vi "HW_Gantner_DLL paths.vi"() -> (2 "DLL paths":T1)   [LabVIEW 2016]
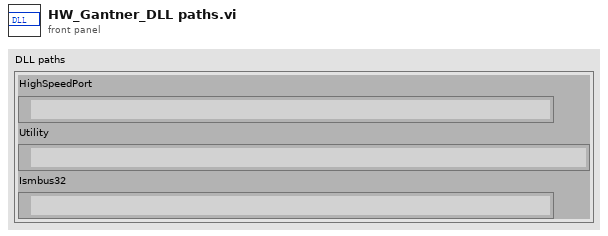
[diagram p1: front panel]
types:
  T1 = cluster{"HighSpeedPort":path, "Utility":path, "Ismbus32":path}
  T2 = enum32{"invalid app kind", "Development System", "Run Time System", "Student Edition", "Embedded LabVIEW", "Evaluation", "Custom"}
  T3 = cluster{"appended path":path, "appended path":path, "appended path":path}
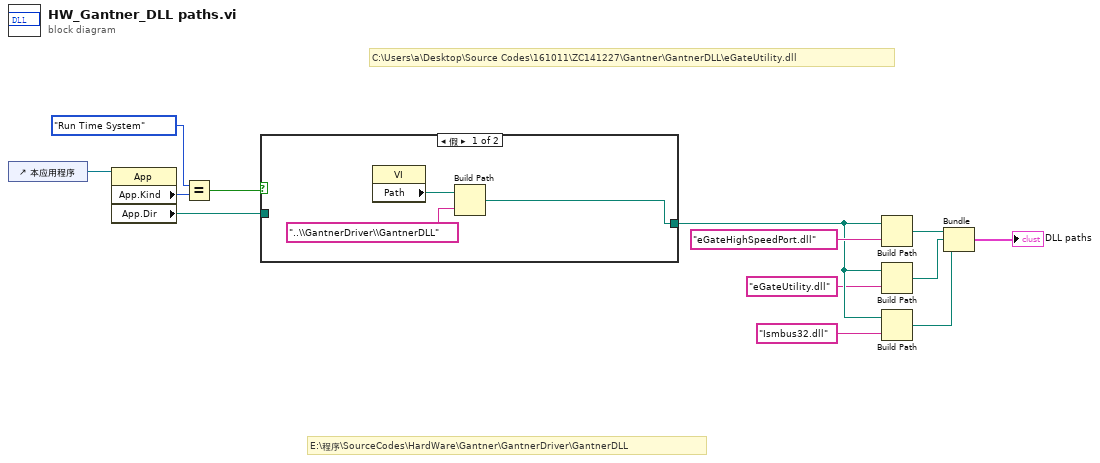
[diagram p0: block diagram]
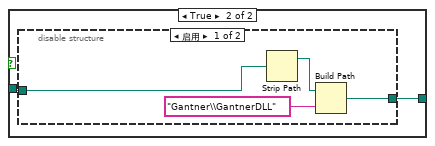
[diagram p2: hidden frame]
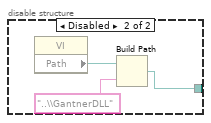
[diagram p3: hidden frame]
diagram:
  # "E:\\程序\\SourceCodes\\HardWare\\Gantner\\GantnerDriver\\GantnerDLL"
  # "C:\\Users\\a\\Desktop\\Source Codes\\161011\\ZC141227\\Gantner\\GantnerDLL\\eGateUtility.dll"
  n1 = control-ref of="本应用程序"() -> (w13:refnum<vi>)
  n2 = property class="App"(reference=w13) -> ("App.Kind"=w12:T2, "App.Dir"=w10:path)  [unwired: 1 in, 2 out]
  n3 = Equal?(x=T2."Run Time System" ("应用程序:类别"), y=w12) -> (x = y?=w1:bool)
  n4 = case shown="假" w1 {
    tunnel: [w14 w17] -> w8
    tunnel: w10 -> [_ w18]
    frame False {
      n5 = property class="VI"() -> ("Path"=w16:path)  [unwired: 2 in, 2 out]
      n6 = Build Path(base path=w16, name or relative path="..\\GantnerDriver\\GantnerDLL" ("名称或相对路径")) -> (appended path=w14:path)
    }
    frame True {
      n7 = disable-structure shown="启用" {
        disable-tunnel: w18 -> [w20 _]
        disable-tunnel: [w21 w23] -> w17
        frame Enabled {
          n8 = Strip Path(path=w20) -> (stripped path=w19:path)  [unwired: 1 out]
          n9 = Build Path(base path=w19, name or relative path="Gantner\\GantnerDLL" ("名称或相对路径")) -> (appended path=w21:path)
        }
        frame Disabled {
          n10 = property class="VI"() -> ("Path"=w25:path)  [unwired: 2 in, 2 out]
          n11 = Build Path(base path=w25, name or relative path="..\\GantnerDLL" ("名称或相对路径")) -> (appended path=w23:path)
        }
      }
    }
  }
  n12 = Build Path(base path=w8, name or relative path="eGateHighSpeedPort.dll" ("名称或相对路径")) -> (appended path=w5:path)
  n13 = Build Path(base path=w8, name or relative path="eGateUtility.dll" ("名称或相对路径")) -> (appended path=w4:path)
  n14 = Build Path(base path=w8, name or relative path="Ismbus32.dll" ("名称或相对路径")) -> (appended path=w3:path)
  n15 = Bundle("appended path"=w5, "appended path"=w4, "appended path"=w3) -> (→"DLL paths":T3)  [unwired: 1 in]
